vi "Parse Frame Config Data.vi"(8 "error in (no error)":errorcluster, 11 "all rows":string[][](array[string])) -> (0 "error out":errorcluster, 3 "SPI FRM Config out":T1[](array[typedef]) {"Addr" format="%x"; "Data" format="%x"})   [LabVIEW 2018, in "Config_Read_SPI.lvclass"]
uses:
  Config_Read_SPI.lvclass
  SPI_FRM_Config.ctl
  Classes/Config_Read/RW_Option.ctl
  SPI_Mode.ctl
  Classes/Config_Read/Config_Read_BML.lvclass
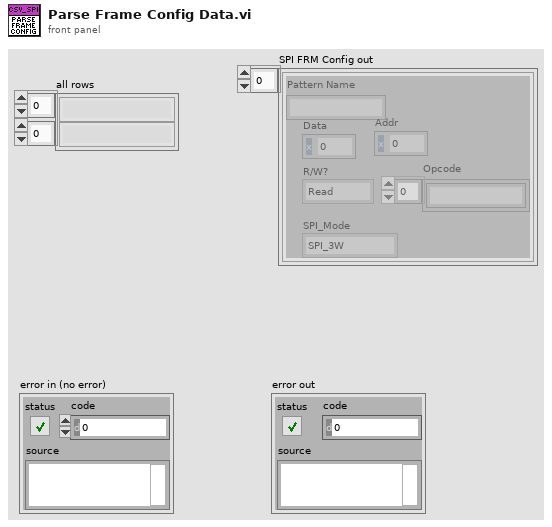
[diagram p1: front panel]
types:
  T1 = typedef "Config_Read_SPI.lvclass/SPI_FRM_Config.ctl" = cluster{"Pattern Name":string, "Data":u16, "Addr":u16, "R/W?":T2, "Opcode":string[], "SPI_Mode":T3}
  T2 = typedef "Config_Read_BML.lvclass/RW_Option.ctl" = enum16{"Read", "Write", "R/W"}
  T3 = typedef "Config_Read_SPI.lvclass/SPI_Mode.ctl" = enum16{"SPI_3W", "SPI_4W"}
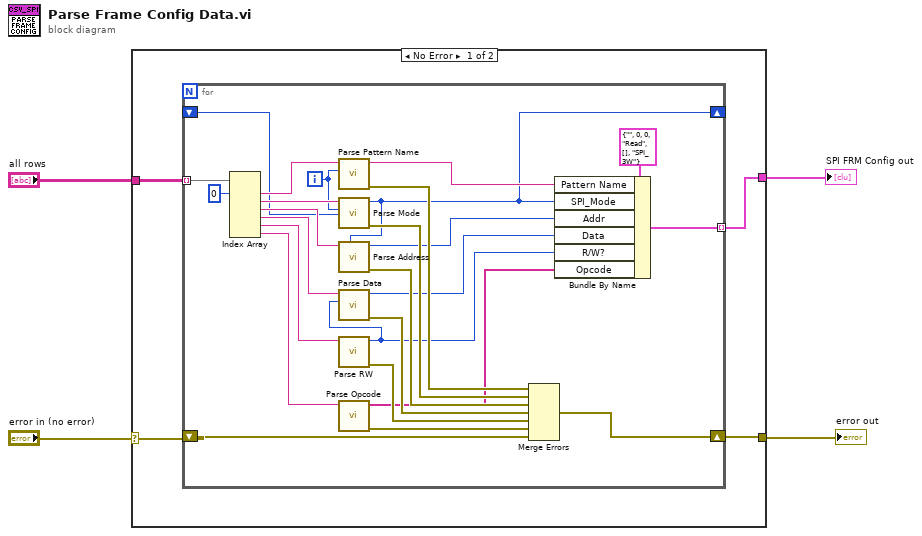
[diagram p0: block diagram]
diagram:
  n1 = case shown="No Error" "error in (no error)" {
    selector: "error in (no error)" -> [w7 w35]
    tunnel: "all rows" -> [w8 _]
    tunnel: [w6 w35] -> w2
    tunnel: [w5 _] -> w1
    frame No Error {
      n2 = for {
        tunnel: w8 -> [w34] mode=indexing
        shift-right: [w32] -> w6
        shift-left: w7 -> [w13]
        tunnel: [w31] -> w5 mode=indexing
        shift-right: [w9] -> _
        shift-left: _ -> [w11]
        i -> [w24]
        n3 = Index Array(array=w34, index #1=0 ("index")) -> (element #1=w30:string, element #2=w25:string, element #3=w23:string, element #4=w21:string, element #5=w18:string, element #6=w15:string)  [unwired: 5 in]
        n4 = call "Parse Pattern Name.vi"("Index"=w24, "Pattern Name"=w30) -> ("error out"=w29:errorcluster, "Pattern Name out"=w28:string)  [unwired: 8 in]
        n5 = call "Parse Mode.vi"("SPI_Mode In"=w11, "index"=w24, "Mode"=w25) -> ("error out"=w26:errorcluster, "SPI_Mode"=w9:T3)  [unwired: 7 in]
        n6 = call "Parse Address.vi"("SPI_Mode"=w9, "Addr in"=w23) -> ("error out"=w22:errorcluster, "Addr out"=w10:u16)  [unwired: 8 in]
        n7 = call "Parse RW.vi"("R/W mode in"=w18) -> ("error out"=w16:errorcluster, "R/W?"=w17:T2)  [unwired: 9 in]
        n8 = call "Parse Data.vi"("R/W?"=w17, "Data in"=w21) -> ("error out"=w19:errorcluster, "Data out"=w20:u16)  [unwired: 8 in]
        n9 = call "Parse Opcode.vi"("Opcode"=w15) -> ("Error out"=w14:errorcluster, "Opcode Array"=w12:string[])  [unwired: 9 in]
        n10 = Merge Errors(w29, w26, w22, w19, w16, w14, w13) -> (w32:errorcluster)
        n11 = Bundle By Name(cluster=T1 {"Pattern Name"="", "Data"=0, "Addr"=0, "R/W?"=enum."Read", "Opcode"=[], "SPI_Mode"=enum."SPI_3W"} ("SPI_FRM_Config"), "Pattern Name"=w28, "SPI_Mode"=w9, "Addr"=w10, "Data"=w20, "R/W?"=w17, "Opcode"=w12) -> (w31:T1)
      }
    }
    frame Error {
    }
  }
  "error out" <- w2
  "SPI FRM Config out" <- w1
